vi "OmniDyn2ROS.vi"(9 "omni_dyn":T1, 10 "frame_id":string, 11 "msg in":string) -> (3 "msg out":string)   [LabVIEW 2014]
uses:
  <vilib>/robotics/TaimiOmni/TaimiOmni/TaimiOmniVelocity.ctl
  <userlib>/ROS for LabVIEW Software/ROS/MessageBuilding/std_msgs/subs/float64Scalar.vi
  <vilib>/robotics/TaimiOmni/TaimiOmni/TaimiOmni.lvclass
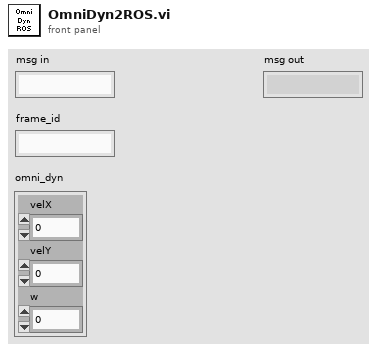
[diagram p1: front panel]
types:
  T1 = typedef "TaimiOmni.lvclass/TaimiOmniVelocity.ctl" = cluster{"velX":dbl, "velY":dbl, "w":dbl}
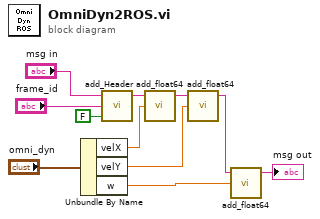
[diagram p0: block diagram]
diagram:
  n1 = Unbundle By Name("omni_dyn") -> ("velX"=w6:dbl, "velY"=w4:dbl, "w"=w2:dbl)
  n2 = call <userlib>:"add_Header.vi"("reset seq?"=FALSE, "frame_id"="frame_id", "msg in"="msg in") -> ("msg out"=w7:string)  [unwired: 2 in]
  n3 = call-poly <userlib>:"add_float64.vi"("Numeric"=w6, "msg in"=w7) -> ("msg out"=w5:string)  [unwired: 3 in]
  n4 = call-poly <userlib>:"add_float64.vi"("Numeric"=w4, "msg in"=w5) -> ("msg out"=w3:string)  [unwired: 3 in]
  n5 = call-poly <userlib>:"add_float64.vi"("Numeric"=w2, "msg in"=w3) -> ("msg out"=→"msg out":string)  [unwired: 3 in]
